vi "jump.vi"(1 "times":i32, 3 "yo":i32) -> (0 "y":i32)   [LabVIEW 2014]
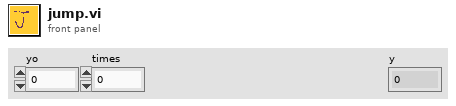
[diagram p1: front panel]
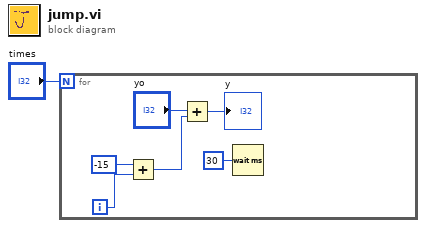
[diagram p0: block diagram]
diagram:
  n1 = for {
    N: "times" -> [_]
    i -> [w7]
    n2 = Add(x=-15, y=w7) -> (x+y=w5:i32)
    n3 = Add(x="yo", y=w5) -> (x+y=→"y":i32)
    n4 = Wait (ms)(milliseconds to wait=u32 30) -> ()  [unwired: 1 out]
  }
